vi "core_persist_controls_auto.vi"(7 "action":T1, 8 "error in":errorcluster, 10 "crtl refs in":refnum<vi>[](array[refnum])) -> (0 "error out":errorcluster, 2 "ctrl refs out":refnum<vi>[](array[refnum]))   [LabVIEW 2015, in "_persist_controls_polys.lvlib"]
doc: "Writes the values of an array of controls to a configuration file or reads them back.\n<b>Control References</b> is an array of the references of the controls to be saved.\n\nThe configuration file is named after the VI the first control in the array is in and is saved in the LabVIEW Data folder"
uses:
  _persist_controls_polys.lvlib
  Actions.ctl
  <vilib>/Utility/config.llb/NI_LVConfig.lvlib
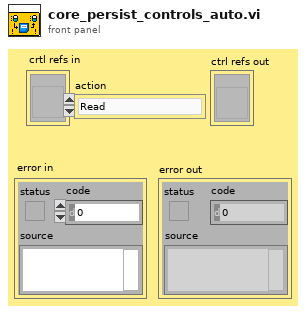
[diagram p1: front panel]
types:
  T1 = typedef "Actions.ctl" = enum16{"Read", "Write", "Read and Create"}
  T2 = typedef "NI_LVConfig.lvlib/Config Data RefNum.ctl" = refnum<k1>
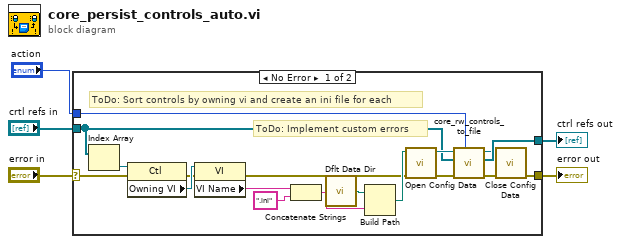
[diagram p0: block diagram]
diagram:
  n1 = case shown="No Error" "error in" {
    selector: "error in" -> [w11 w25]
    tunnel: "action" -> [w6 _]
    tunnel: "crtl refs in" -> [w7 w24]
    tunnel: [w8 w25] -> w3
    tunnel: [w23 w24] -> w2
    frame No Error {
      # "ToDo: Implement custom errors"
      # "ToDo: Sort controls by owning vi and create an ini file for each"
      n2 = Index Array(array=w7) -> (element=w13:refnum<vi>)  [unwired: 1 in]
      n3 = property class="Ctl"(reference=w13, error in=w11) -> (error out=w10:errorcluster, "Owning VI"=w12:refnum<vi>)  [unwired: 1 out]
      n4 = property class="VI"(reference=w12, error in=w10) -> (error out=w9:errorcluster, "VI Name"=w19:string)  [unwired: 1 out]
      n5 = Concatenate Strings(w19, ".ini" ("string")) -> (w21:string)
      n6 = call <vilib>:"Dflt Data Dir.vi"() -> ("App:Default Data Directory"=w20:path)
      n7 = Build Path(base path=w20, name or relative path=w21) -> (appended path=w14:path)
      n8 = call <vilib>:"Open Config Data.vi"("error in (no error)"=w9, "configuration file path"=w14) -> ("error out"=w15:errorcluster, "refnum"=w17:T2)  [unwired: 7 in, 1 out]
      n9 = call "core_rw_controls_to_file.vi"("Action"=w6, "error in"=w15, "ctrl refs in"=w7, "config ref"=w17) -> ("error out"=w18:errorcluster, "ctrl refs out"=w23:refnum<vi>[], "config ref duplicate"=w16:T2)  [unwired: 5 in]
      n10 = call <vilib>:"Close Config Data.vi"("error in (no error)"=w18, "refnum"=w16) -> ("error out"=w8:errorcluster)  [unwired: 8 in, 1 out]
    }
    frame Error {
    }
  }
  "error out" <- w3
  "ctrl refs out" <- w2
